vi "Preprocessing.vi"() -> (1 "TimeStamp":dbl[](graph), 4 "Potência Ativa A 3":dbl[](graph), 7 "Potência Ativa A 2":dbl[](graph), 9 "Potência Ativa A":dbl[](graph))   [LabVIEW 2024]
uses:
  <vilib>/numeric/Random Number (Range) DBL.vi
panel:
  out "Potencai Ativa A 3":dbl[](array[numeric])
  out "Corrente A 3":dbl[](array[numeric])
  out "Tensão A 3":dbl[](array[numeric])
  out "Potencai Ativa A 2":dbl[](array[numeric])
  out "Corrente A 2":dbl[](array[numeric])
  out "Tensão A 2":dbl[](array[numeric])
  out "Potencai Ativa A":dbl[](array[numeric])
  out "Corrente A":dbl[](array[numeric])
  out "Tensão A":dbl[](array[numeric])
  out "Fator de potência":dbl
  in  "Limite inferior FP":dbl
  in  "Limite Superior FP":dbl=100.0
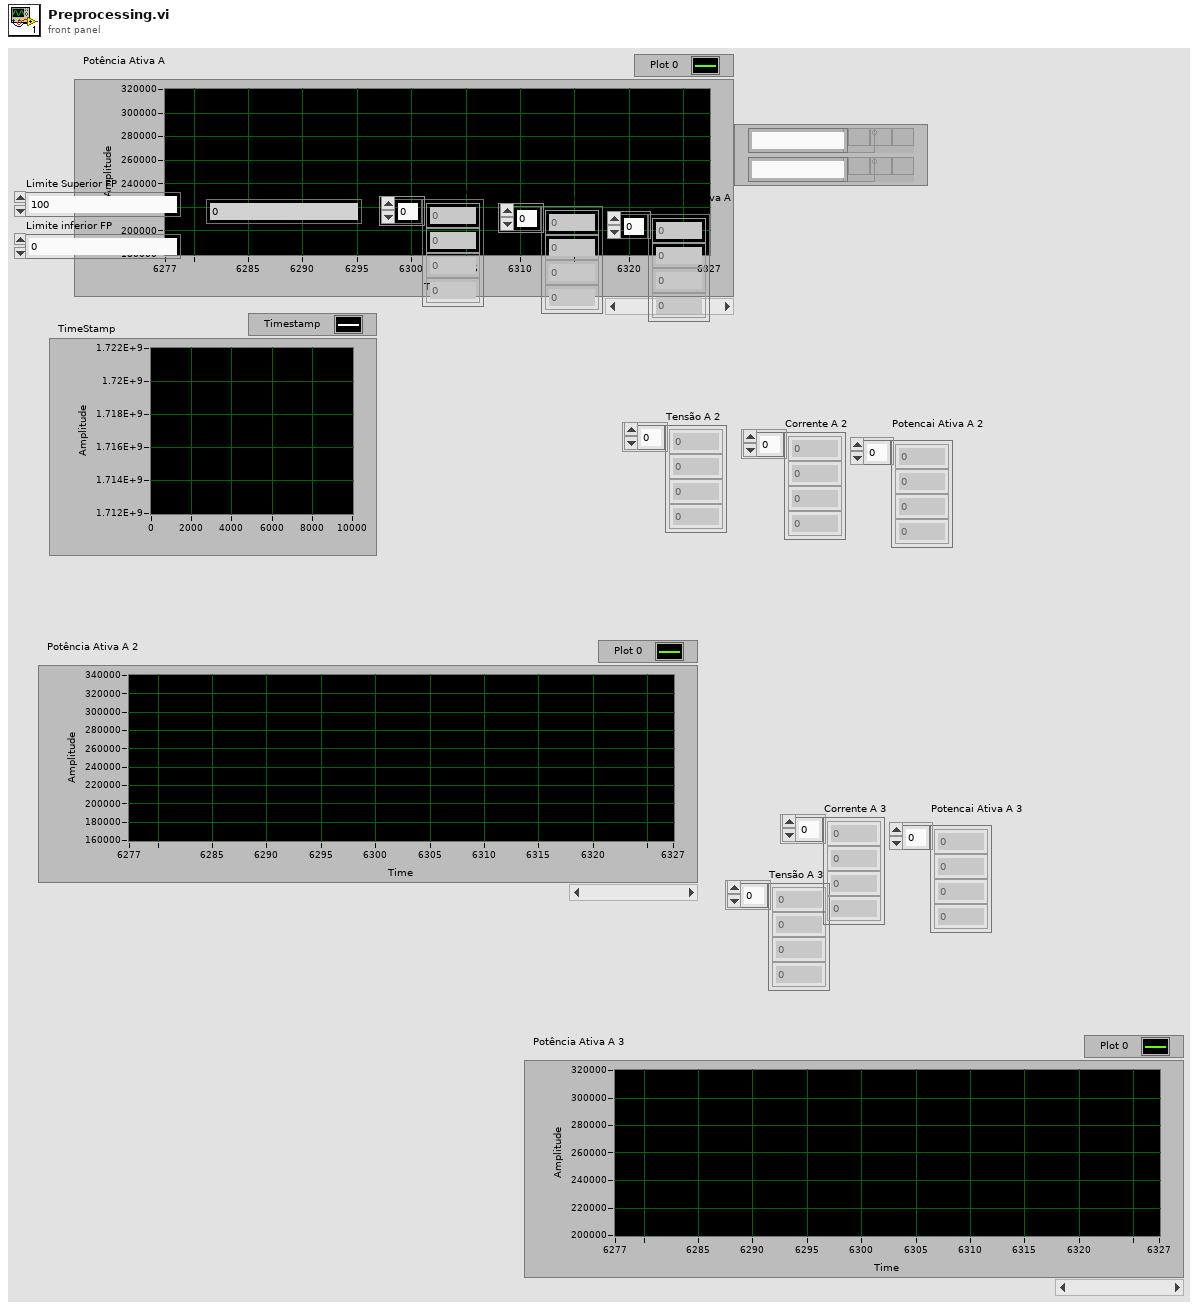
[diagram p1: front panel]
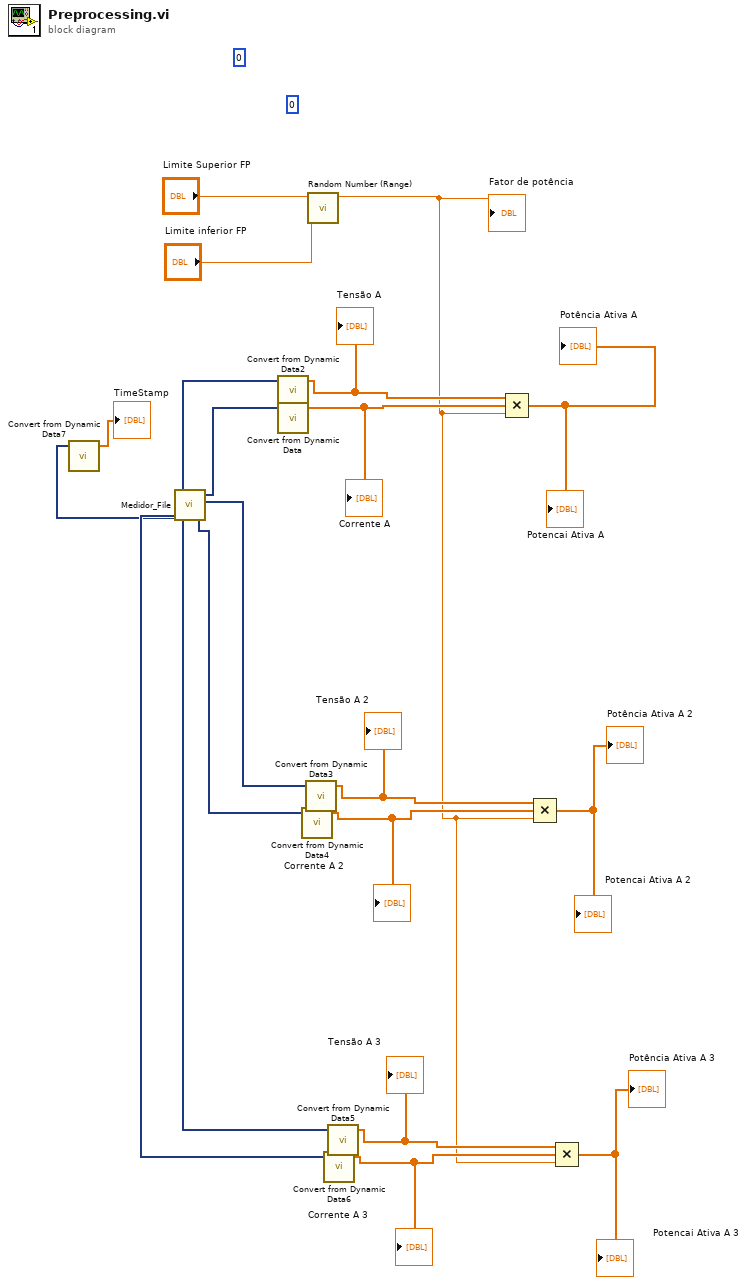
[diagram p0: block diagram]
diagram:
  (unwired) 0
  (unwired) 0
  n1 = call "Medidor_File.vi"() -> ("Corrente Fase C"=w4:dynamicdata, "Corrente Fase B"=w6:dynamicdata, "Corrente Fase A"=w20:dynamicdata, "TimeStamp"=w2:dynamicdata, "Tensão Fase C"=w3:dynamicdata, "Tensão Fase B"=w5:dynamicdata, "Tensão Fase A"=w19:dynamicdata)
  n2 = call "Convert from Dynamic Data7"("Dynamic Data Type"=w2) -> ("Array"=→"TimeStamp":dbl[])  [unwired: 3 in]
  n3 = call "Convert from Dynamic Data2"("Dynamic Data Type"=w19) -> ("Array"=w18:dbl[])  [unwired: 3 in]
  "Tensão A" <- w18
  n4 = call "Convert from Dynamic Data"("Dynamic Data Type"=w20) -> ("Array"=w17:dbl[])  [unwired: 3 in]
  "Corrente A" <- w17
  n5 = call "Convert from Dynamic Data4"("Dynamic Data Type"=w6) -> ("Array"=w12:dbl[])  [unwired: 3 in]
  "Corrente A 2" <- w12
  n6 = call "Convert from Dynamic Data3"("Dynamic Data Type"=w5) -> ("Array"=w13:dbl[])  [unwired: 3 in]
  "Tensão A 2" <- w13
  n7 = call-poly <vilib>:"Random Number (Range).vi"("lower bound (0)"="Limite inferior FP", "upper bound (100)"="Limite Superior FP") -> ("number"=w7:dbl)  [unwired: 9 in]
  "Fator de potência" <- w7
  n8 = call "Convert from Dynamic Data6"("Dynamic Data Type"=w4) -> ("Array"=w9:dbl[])  [unwired: 3 in]
  "Corrente A 3" <- w9
  n9 = call "Convert from Dynamic Data5"("Dynamic Data Type"=w3) -> ("Array"=w10:dbl[])  [unwired: 3 in]
  "Tensão A 3" <- w10
  n10 = Compound Arithmetic op=MULTIPLY(w18, w17, w7) -> (→"Potência Ativa A" →"Potencai Ativa A":dbl[])
  n11 = Compound Arithmetic op=MULTIPLY(w13, w12, w7) -> (→"Potência Ativa A 2" →"Potencai Ativa A 2":dbl[])
  n12 = Compound Arithmetic op=MULTIPLY(w10, w9, w7) -> (→"Potência Ativa A 3" →"Potencai Ativa A 3":dbl[])
